vi "Association Retrieve Record.vi"(8 "error in (no error)":errorcluster, 11 "Statement Refnum":T1) -> (0 "error out":errorcluster, 2 "Association":T2, 3 "Statement Refnum":T1)   [LabVIEW 2011]
uses:
  Association Record.ctl
  SI.LIB/ODBC/SQL Controls/Statement Refnum.ctl
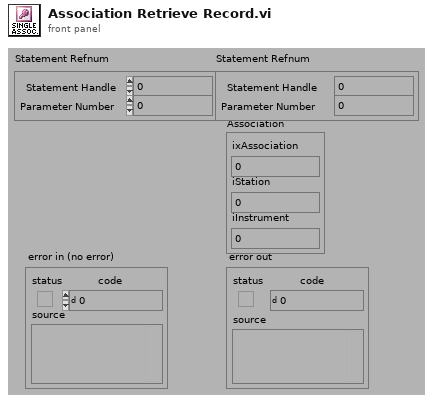
[diagram p1: front panel]
types:
  T1 = typedef "Statement Refnum.ctl" = cluster{"Statement Handle":i32, "Parameter Number":u16}
  T2 = typedef "Association Record.ctl" = cluster{"ixAssociation":i32, "iStation":i32, "iInstrument":i32}
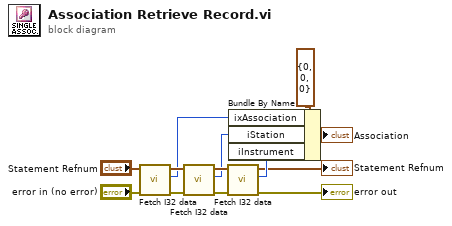
[diagram p0: block diagram]
diagram:
  n1 = call "Fetch I32 data.vi"("error in (no error)"="error in (no error)", "Statement Refnum"="Statement Refnum") -> ("error out"=w11:errorcluster, "Data"=w7:i32, "Statement Refnum"=w10:T1)  [unwired: 3 out]
  n2 = call "Fetch I32 data.vi"("error in (no error)"=w11, "Statement Refnum"=w10) -> ("error out"=w8:errorcluster, "Data"=w6:i32, "Statement Refnum"=w9:T1)  [unwired: 3 out]
  n3 = call "Fetch I32 data.vi"("error in (no error)"=w8, "Statement Refnum"=w9) -> ("error out"=→"error out":errorcluster, "Data"=w5:i32, "Statement Refnum"=→"Statement Refnum":T1)  [unwired: 3 out]
  n4 = Bundle By Name(cluster=T2 {"ixAssociation"=0, "iStation"=0, "iInstrument"=0} ("Association Record"), "ixAssociation"=w7, "iStation"=w6, "iInstrument"=w5) -> (→"Association":T2)
